vi "CAENHV Get Ch Name.vi"(7 "ChNum":u16, 8 "error in (no error)":errorcluster, 9 "ChList":u16[](array[numeric]), 10 "slot":u16, 11 "handle":i32) -> (0 "error out":errorcluster, 3 "ChNameList":string[](array[string]))   [LabVIEW 2018, in "CAENHVWrapper.lvlib"]
doc: "CAENHVLIB_API CAENHVRESULT CAENHV_GetChName(int handle, ushort slot, \n ushort ChNum, const ushort *ChList, char (*ChNameList)[MAX_CH_NAME]);"
uses:
  <instrlib>/CAENHVWrapper/CAENHVWrapper.lvlib
  <instrlib>/CAENHVWrapper/VIs/CAENHVWrapper.dll
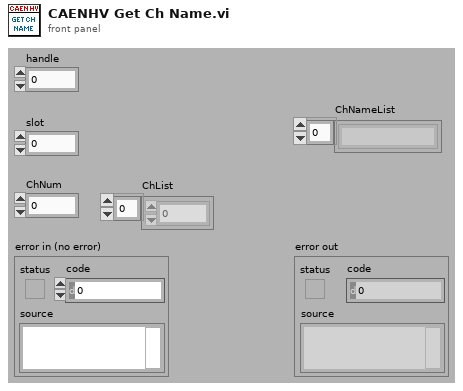
[diagram p1: front panel]
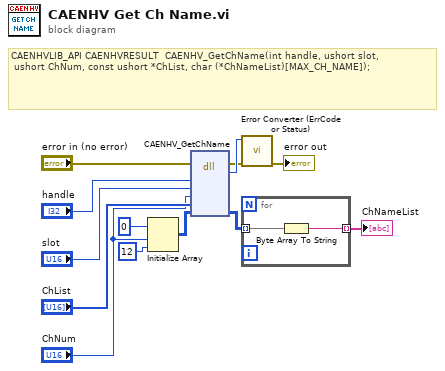
[diagram p0: block diagram]
diagram:
  # "CAENHVLIB_API CAENHVRESULT  CAENHV_GetChName(int handle, ushort slot, \n ushort ChNum, const ushort *ChList, char (*ChNameList)[MAX_CH_NAME]);"
  n1 = Initialize Array(u8 0 ("element"), "ChNum", 12 ("dimension size")) -> (w4:u8[][])
  n2 = dll-call lib="C:/Program Files (x86)/National Instruments/LabVIEW 2018/instr.lib/CAENHVWrapper/VIs/CAENHVWrapper.*" fn="CAENHV_GetChName"(error in="error in (no error)", "handle"="handle", "slot"="slot", "ChNum"="ChNum", "ChList"="ChList", "ChNameList"=w4) -> (error out=w9:errorcluster, "return type"=w10:i32, "ChNameList"=w3:u8[][])  [unwired: 6 in, 1 out]
  n3 = call <instrlib>:"Error Converter (ErrCode or Status).vi"("error in (no error)"=w9, "error code"=w10) -> ("error out"=→"error out":errorcluster)  [unwired: 9 in]
  n4 = for {
    tunnel: [w15] -> w6 mode=indexing
    tunnel: w3 -> [w14] mode=indexing
    n5 = Byte Array To String(unsigned byte array=w14) -> (string=w15:string)
  }
  "ChNameList" <- w6
